vi "Flow Read.vi"   [LabVIEW 2023, in "Chiller.lvclass"]
uses:
  Chiller.lvclass
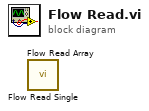
[diagram p0: block diagram]
diagram:
  n1 = call "Flow Read Single.vi"() -> ()  [unwired: 8 in, 4 out]
  n2 = call "Flow Read Array.vi"() -> ()  [unwired: 8 in, 4 out]
